vi "convert to TDMS.vi"(7 "defrag?":bool=TRUE, 8 "error in":errorcluster, 11 "path":path) -> (0 "error out":errorcluster)   [LabVIEW 2013, in "Binary datalogger runtime.lvclass"]
uses:
  Binary datalogger runtime.lvclass
  <vilib>/NI/Tag Bus/tag/count types.vi
  <vilib>/NI/Tag Bus/tag/index to type.vi
  <vilib>/NI/Tag Bus/tag/tag descriptor.lvclass
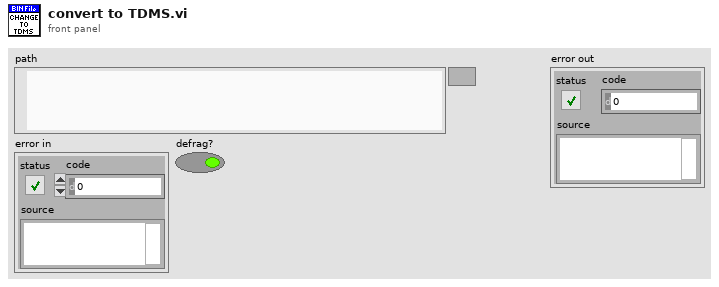
[diagram p1: front panel]
types:
  T1 = typedef "Binary datalogger runtime.lvclass/data cache.ctl" = cluster{"timestamps":timestamp[], "dataset":T2[]}
  T2 = typedef "tag bus.lvlib/data table.lvlib/data table.ctl" = cluster{"Double":dbl[], "Single":sgl[], "I64":i64[], "I32":i32[], "I16":i16[], "I8":i8[], "U64":u64[], "U32":u32[], "U16":u16[], "U8":u8[], "Boolean":bool[], "String":string[], "Array of Double":cluster{"DBL Array":dbl[]}[], "Array of Single":cluster{"SGL Array":sgl[]}[], "Array of I64":cluster{"I64 Array":i64[]}[], "Array of I32":cluster{"I32 Array":i32[]}[], "Array of I16":cluster{"I16 Array":i16[]}[], "Array of I8":cluster{"I8 Array":i8[]}[], "Array of U64":cluster{"U64 Array":u64[]}[], "Array of U32":cluster{"U32 Array":u32[]}[], "Array of U16":cluster{"U16 Array":u16[]}[], "Array of U8":cluster{"U8 Array":u8[]}[], "Array of Boolean":cluster{"Boolean Array":bool[]}[], "Array of String":cluster{"String Array":string[]}[]}
  T3 = typedef "tag bus.lvlib/data dictionary.lvclass/full data dictionary.ctl" = cluster{"Double":string[], "Single":string[], "I64":string[], "I32":string[], "I16":string[], "I8":string[], "U64":string[], "U32":string[], "U16":string[], "U8":string[], "Boolean":string[], "String":string[], "Array of Double":string[], "Array of Single":string[], "Array of I64":string[], "Array of I32":string[], "Array of I16":string[], "Array of I8":string[], "Array of U64":string[], "Array of U32":string[], "Array of U16":string[], "Array of U8":string[], "Array of Boolean":string[], "Array of String":string[]}
  T4 = enum16{"open", "open or create", "create or replace", "create", "open (read-only)"}
  T5 = typedef "tag bus.lvlib/tag descriptor.lvclass/Data Type.ctl" = enum16{"Double", "Single", "I64", "I32", "I16", "I8", "U64", "U32", "U16", "U8", "Boolean", "String", "Array of Double", "Array of Single", "Array of I64", "Array of I32", "Array of I16", "Array of I8", "Array of U64", "Array of U32", "Array of U16", "Array of U8", "Array of Boolean", "Array of String"}
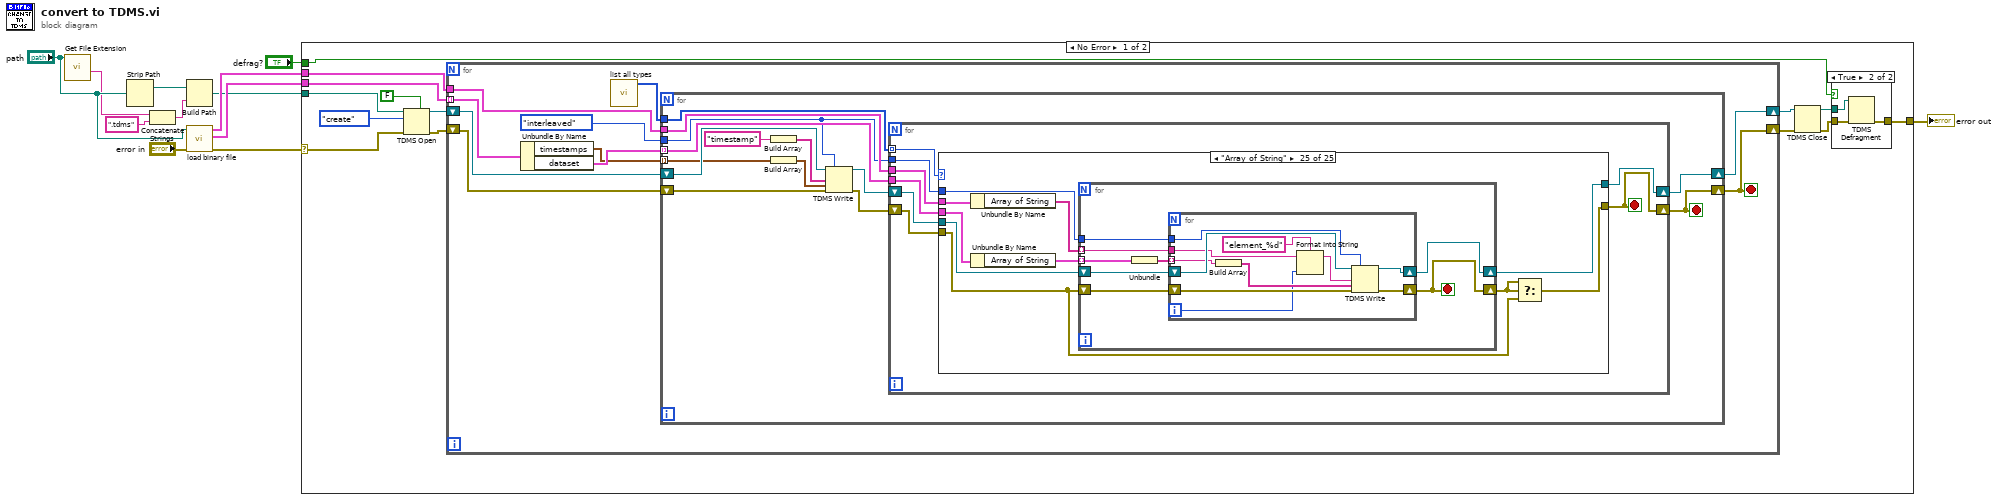
[diagram p0: block diagram]
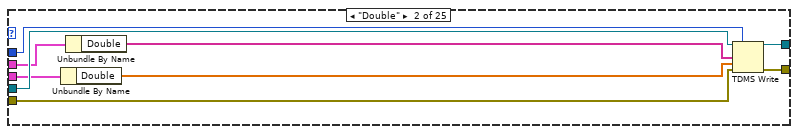
[diagram p3: hidden frame]
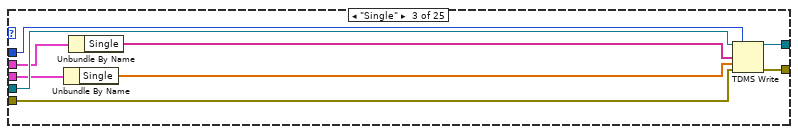
[diagram p4: hidden frame]
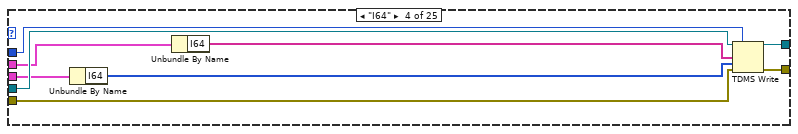
[diagram p5: hidden frame]
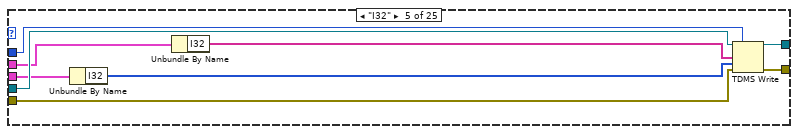
[diagram p6: hidden frame]
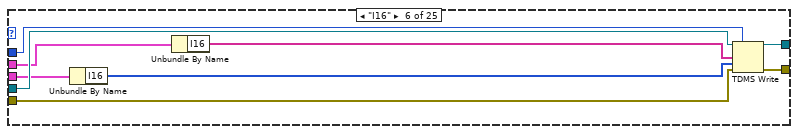
[diagram p7: hidden frame]
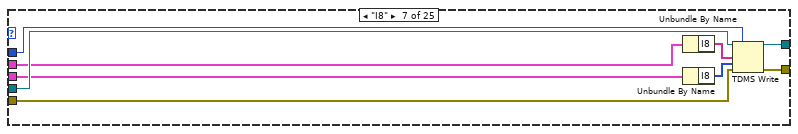
[diagram p8: hidden frame]
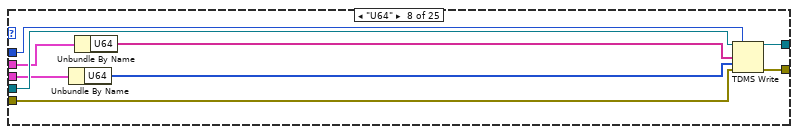
[diagram p9: hidden frame]
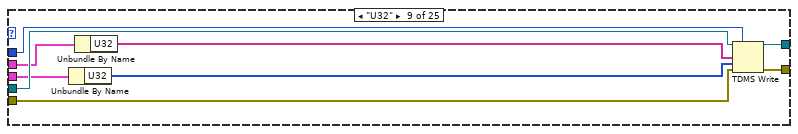
[diagram p10: hidden frame]
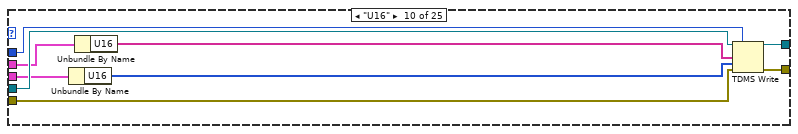
[diagram p11: hidden frame]
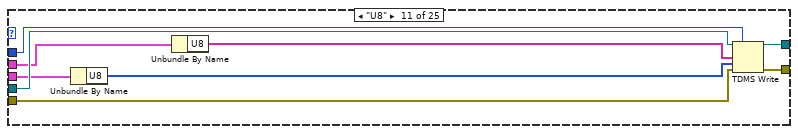
[diagram p12: hidden frame]
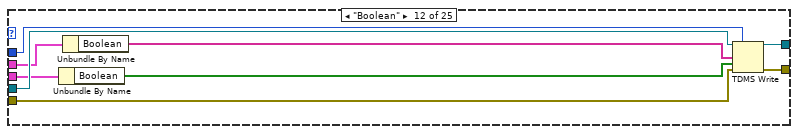
[diagram p13: hidden frame]
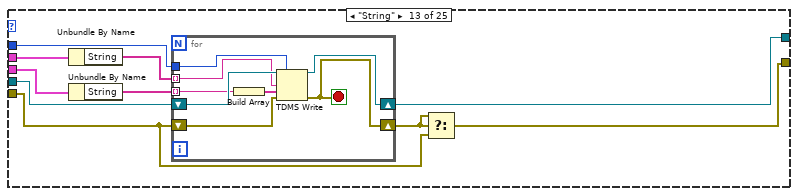
[diagram p14: hidden frame]
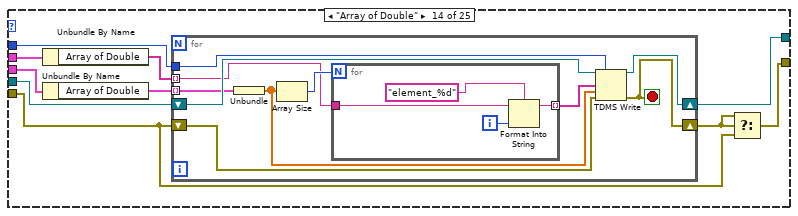
[diagram p15: hidden frame]
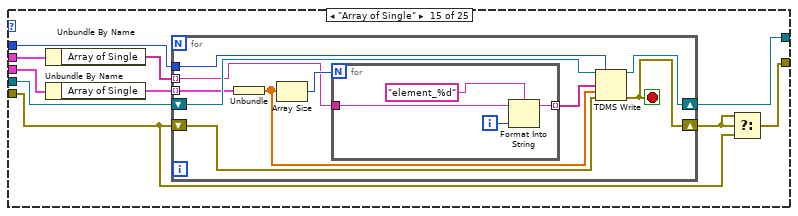
[diagram p16: hidden frame]
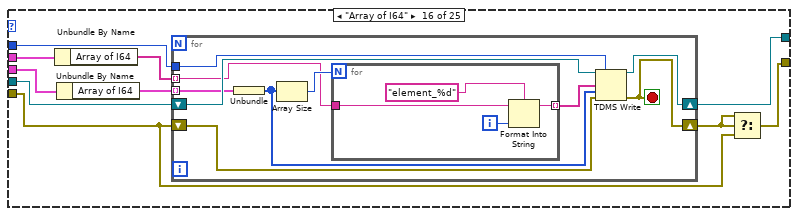
[diagram p17: hidden frame]
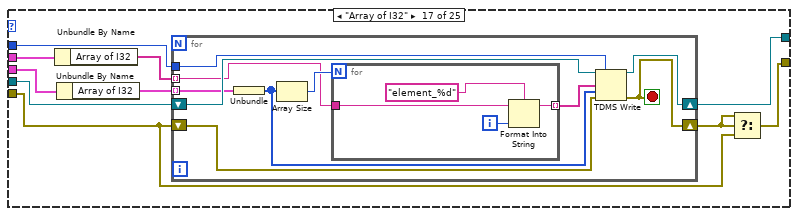
[diagram p18: hidden frame]
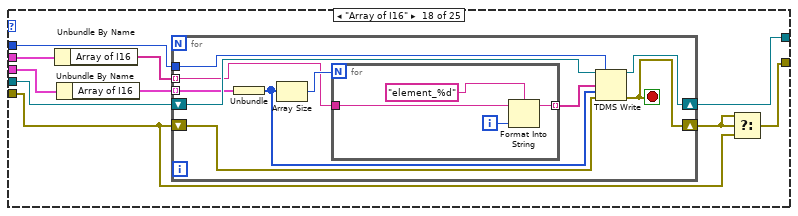
[diagram p19: hidden frame]
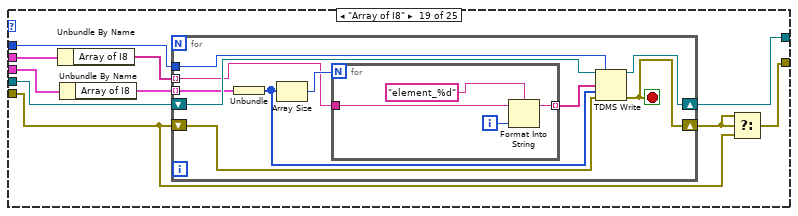
[diagram p20: hidden frame]
diagram:
  n1 = call <vilib>:"Get File Extension.vi"("file"="path") -> ("filename without extension"=w6:string)  [unwired: 7 in, 3 out]
  n2 = Strip Path(path="path") -> (stripped path=w4:path)  [unwired: 1 out]
  n3 = Concatenate Strings(w6, ".tdms" ("string")) -> (w3:string)
  n4 = Build Path(base path=w4, name or relative path=w3) -> (appended path=w2:path)
  n5 = call "load binary file.vi"("error in"="error in", "path"="path") -> ("error out"=w11:errorcluster, "data"=w9:T1[], "dictionary"=w8:T3)  [unwired: 5 in, 2 out]
  n6 = case shown="No Error" w11 {
    selector: w11 -> [w26 w475]
    tunnel: [w21 w475] -> w10
    tunnel: w9 -> [w14 _]
    tunnel: w8 -> [w13 _]
    tunnel: w2 -> [w25 _]
    tunnel: "defrag?" -> [w19 _]
    frame No Error {
      n7 = TDMS Open(5:FALSE ("create index file? (T)"), 8:w26, 10:T4."create" ("operation (0:open)"), 11:w25) -> (0:w16:errorcluster, 3:w18:refnum<k34>)  [unwired: 3 in]
      n8 = for {
        shift-right: [w36] -> w17
        shift-left: w18 -> [w30]
        shift-right: [w35] -> w15
        shift-left: w16 -> [w31]
        tunnel: w14 -> [w34] mode=indexing
        tunnel: w13 -> [w32]
        stop <- w35 stop-if-true
        n9 = Unbundle By Name(w34) -> ("timestamps"=w27:timestamp[], "dataset"=w33:T2[])
        n10 = call <vilib>:"list all types.vi"() -> ("all types"=w29:T5[])  [unwired: 11 in]
        n11 = for {
          shift-right: [w49] -> w36
          shift-left: w30 -> [w43]
          shift-right: [w45] -> w35
          shift-left: w31 -> [w48]
          tunnel: w33 -> [w46] mode=indexing
          tunnel: w32 -> [w47]
          tunnel: w29 -> [w50]
          tunnel: enum16{"decimated", "interleaved"}."interleaved" ("data layout (0:decimated)") -> [w41]
          tunnel: w27 -> [w38] mode=indexing
          stop <- w45 stop-if-true
          n12 = Build Array("timestamp") -> (w39:string[])
          n13 = Build Array(w38) -> (w37:timestamp[])
          n14 = TDMS Write(0:w43, 1:w41, 7:w39, 9:w37, 11:w48) -> (4:w42:refnum<k34>, 15:w44:errorcluster)  [unwired: 1 in, 2 out]
          n15 = for {
            tunnel: w50 -> [w58] mode=indexing
            tunnel: w47 -> [w54]
            tunnel: w46 -> [w53]
            tunnel: w41 -> [w52]
            shift-right: [w57] -> w49
            shift-left: w42 -> [w56]
            shift-right: [w51] -> w45
            shift-left: w44 -> [w55]
            stop <- w51 stop-if-true
            n16 = case shown="\"Array of String\"" w58 {
              tunnel: [w60 w66 w75 w84 w93 w102 w111 w120 w129 w138 w147 w156 w168 w186 w210 w234 w258 w282 w306 w330 w354 w378 w402 w426 w450] -> w57
              tunnel: w56 -> [w60 w69 w78 w87 w96 w105 w114 w123 w132 w141 w150 w159 w169 w187 w211 w235 w259 w283 w307 w331 w355 w379 w403 w427 w451]
              tunnel: w55 -> [w59 w68 w77 w86 w95 w104 w113 w122 w131 w140 w149 w158 w161 w179 w203 w227 w251 w275 w299 w323 w347 w371 w395 w419 w443]
              tunnel: [w59 w67 w76 w85 w94 w103 w112 w121 w130 w139 w148 w157 w160 w178 w202 w226 w250 w274 w298 w322 w346 w370 w394 w418 w442] -> w51
              tunnel: w54 -> [_ w65 w74 w83 w92 w101 w110 w119 w128 w137 w146 w155 w167 w185 w209 w233 w257 w281 w305 w329 w353 w377 w401 w425 w449]
              tunnel: w53 -> [_ w64 w73 w82 w91 w100 w109 w118 w127 w136 w145 w154 w166 w184 w208 w232 w256 w280 w304 w328 w352 w376 w400 w424 w448]
              tunnel: w52 -> [_ w61 w70 w79 w88 w97 w106 w115 w124 w133 w142 w151 w163 w181 w205 w229 w253 w277 w301 w325 w349 w373 w397 w421 w445]
              frame Default {
              }
              frame "Double" {
                n17 = Unbundle By Name(w64) -> ("Double"=w63:dbl[])
                n18 = Unbundle By Name(w65) -> ("Double"=w62:string[])
                n19 = TDMS Write(0:w69, 1:w61, 7:w62, 9:w63, 11:w68) -> (4:w66:refnum<k34>, 15:w67:errorcluster)  [unwired: 1 in, 2 out]
              }
              frame "Single" {
                n20 = Unbundle By Name(w73) -> ("Single"=w72:sgl[])
                n21 = Unbundle By Name(w74) -> ("Single"=w71:string[])
                n22 = TDMS Write(0:w78, 1:w70, 7:w71, 9:w72, 11:w77) -> (4:w75:refnum<k34>, 15:w76:errorcluster)  [unwired: 1 in, 2 out]
              }
              frame "I64" {
                n23 = Unbundle By Name(w82) -> ("I64"=w81:i64[])
                n24 = Unbundle By Name(w83) -> ("I64"=w80:string[])
                n25 = TDMS Write(0:w87, 1:w79, 7:w80, 9:w81, 11:w86) -> (4:w84:refnum<k34>, 15:w85:errorcluster)  [unwired: 1 in, 2 out]
              }
              frame "I32" {
                n26 = Unbundle By Name(w91) -> ("I32"=w90:i32[])
                n27 = Unbundle By Name(w92) -> ("I32"=w89:string[])
                n28 = TDMS Write(0:w96, 1:w88, 7:w89, 9:w90, 11:w95) -> (4:w93:refnum<k34>, 15:w94:errorcluster)  [unwired: 1 in, 2 out]
              }
              frame "I16" {
                n29 = Unbundle By Name(w100) -> ("I16"=w99:i16[])
                n30 = Unbundle By Name(w101) -> ("I16"=w98:string[])
                n31 = TDMS Write(0:w105, 1:w97, 7:w98, 9:w99, 11:w104) -> (4:w102:refnum<k34>, 15:w103:errorcluster)  [unwired: 1 in, 2 out]
              }
              frame "I8" {
                n32 = Unbundle By Name(w110) -> ("I8"=w107:string[])
                n33 = Unbundle By Name(w109) -> ("I8"=w108:i8[])
                n34 = TDMS Write(0:w114, 1:w106, 7:w107, 9:w108, 11:w113) -> (4:w111:refnum<k34>, 15:w112:errorcluster)  [unwired: 1 in, 2 out]
              }
              frame "U64" {
                n35 = Unbundle By Name(w118) -> ("U64"=w117:u64[])
                n36 = Unbundle By Name(w119) -> ("U64"=w116:string[])
                n37 = TDMS Write(0:w123, 1:w115, 7:w116, 9:w117, 11:w122) -> (4:w120:refnum<k34>, 15:w121:errorcluster)  [unwired: 1 in, 2 out]
              }
              frame "U32" {
                n38 = Unbundle By Name(w127) -> ("U32"=w126:u32[])
                n39 = Unbundle By Name(w128) -> ("U32"=w125:string[])
                n40 = TDMS Write(0:w132, 1:w124, 7:w125, 9:w126, 11:w131) -> (4:w129:refnum<k34>, 15:w130:errorcluster)  [unwired: 1 in, 2 out]
              }
              frame "U16" {
                n41 = Unbundle By Name(w136) -> ("U16"=w135:u16[])
                n42 = Unbundle By Name(w137) -> ("U16"=w134:string[])
                n43 = TDMS Write(0:w141, 1:w133, 7:w134, 9:w135, 11:w140) -> (4:w138:refnum<k34>, 15:w139:errorcluster)  [unwired: 1 in, 2 out]
              }
              frame "U8" {
                n44 = Unbundle By Name(w145) -> ("U8"=w144:u8[])
                n45 = Unbundle By Name(w146) -> ("U8"=w143:string[])
                n46 = TDMS Write(0:w150, 1:w142, 7:w143, 9:w144, 11:w149) -> (4:w147:refnum<k34>, 15:w148:errorcluster)  [unwired: 1 in, 2 out]
              }
              frame "Boolean" {
                n47 = Unbundle By Name(w154) -> ("Boolean"=w153:bool[])
                n48 = Unbundle By Name(w155) -> ("Boolean"=w152:string[])
                n49 = TDMS Write(0:w159, 1:w151, 7:w152, 9:w153, 11:w158) -> (4:w156:refnum<k34>, 15:w157:errorcluster)  [unwired: 1 in, 2 out]
              }
              frame "String" {
                n50 = Unbundle By Name(w167) -> ("String"=w164:string[])
                n51 = Unbundle By Name(w166) -> ("String"=w165:string[])
                n52 = for {
                  tunnel: w165 -> [w174] mode=indexing
                  tunnel: w164 -> [w172] mode=indexing
                  tunnel: w163 -> [w173]
                  shift-right: [w175] -> w168
                  shift-left: w169 -> [w177]
                  shift-right: [w170] -> w162
                  shift-left: w161 -> [w176]
                  stop <- w170 stop-if-true
                  n53 = Build Array(w174) -> (w171:string[])
                  n54 = TDMS Write(0:w177, 1:w173, 7:w172, 9:w171, 11:w176) -> (4:w175:refnum<k34>, 15:w170:errorcluster)  [unwired: 1 in, 2 out]
                }
                n55 = Select(t=w162, s=w162, f=w161) -> (s? t:f=w160:errorcluster)
              }
              frame "Array of Double" {
                n56 = Unbundle By Name(w185) -> ("Array of Double"=w182:string[])
                n57 = Unbundle By Name(w184) -> ("Array of Double"=w183:cluster{"DBL Array":dbl[]}[])
                n58 = for {
                  tunnel: w183 -> [w192] mode=indexing
                  tunnel: w182 -> [w189] mode=indexing
                  tunnel: w181 -> [w194]
                  shift-right: [w195] -> w186
                  shift-left: w187 -> [w197]
                  shift-right: [w193] -> w180
                  shift-left: w179 -> [w196]
                  stop <- w193 stop-if-true
                  n59 = Unbundle(w192) -> ("DBL Array"=w191:dbl[])
                  n60 = Array Size(array=w191) -> (size(s)=w190:i32)
                  n61 = for {
                    N: w190 -> [_]
                    tunnel: w189 -> [w201]
                    tunnel: [w198] -> w188 mode=indexing
                    i -> [w200]
                    n62 = Format Into String(format string="element_%d", initial string=w201, w200) -> (resulting string=w198:string)  [unwired: 1 in, 1 out]
                  }
                  n63 = TDMS Write(0:w197, 1:w194, 7:w188, 9:w191, 11:w196) -> (4:w195:refnum<k34>, 15:w193:errorcluster)  [unwired: 1 in, 2 out]
                }
                n64 = Select(t=w180, s=w180, f=w179) -> (s? t:f=w178:errorcluster)
              }
              frame "Array of Single" {
                n65 = Unbundle By Name(w209) -> ("Array of Single"=w206:string[])
                n66 = Unbundle By Name(w208) -> ("Array of Single"=w207:cluster{"SGL Array":sgl[]}[])
                n67 = for {
                  tunnel: w207 -> [w216] mode=indexing
                  tunnel: w206 -> [w213] mode=indexing
                  tunnel: w205 -> [w218]
                  shift-right: [w219] -> w210
                  shift-left: w211 -> [w221]
                  shift-right: [w217] -> w204
                  shift-left: w203 -> [w220]
                  stop <- w217 stop-if-true
                  n68 = Unbundle(w216) -> ("SGL Array"=w215:sgl[])
                  n69 = Array Size(array=w215) -> (size(s)=w214:i32)
                  n70 = for {
                    N: w214 -> [_]
                    tunnel: w213 -> [w225]
                    tunnel: [w222] -> w212 mode=indexing
                    i -> [w224]
                    n71 = Format Into String(format string="element_%d", initial string=w225, w224) -> (resulting string=w222:string)  [unwired: 1 in, 1 out]
                  }
                  n72 = TDMS Write(0:w221, 1:w218, 7:w212, 9:w215, 11:w220) -> (4:w219:refnum<k34>, 15:w217:errorcluster)  [unwired: 1 in, 2 out]
                }
                n73 = Select(t=w204, s=w204, f=w203) -> (s? t:f=w202:errorcluster)
              }
              frame "Array of I64" {
                n74 = Unbundle By Name(w233) -> ("Array of I64"=w230:string[])
                n75 = Unbundle By Name(w232) -> ("Array of I64"=w231:cluster{"I64 Array":i64[]}[])
                n76 = for {
                  tunnel: w231 -> [w240] mode=indexing
                  tunnel: w230 -> [w237] mode=indexing
                  tunnel: w229 -> [w242]
                  shift-right: [w243] -> w234
                  shift-left: w235 -> [w245]
                  shift-right: [w241] -> w228
                  shift-left: w227 -> [w244]
                  stop <- w241 stop-if-true
                  n77 = Unbundle(w240) -> ("I64 Array"=w239:i64[])
                  n78 = Array Size(array=w239) -> (size(s)=w238:i32)
                  n79 = for {
                    N: w238 -> [_]
                    tunnel: w237 -> [w249]
                    tunnel: [w246] -> w236 mode=indexing
                    i -> [w248]
                    n80 = Format Into String(format string="element_%d", initial string=w249, w248) -> (resulting string=w246:string)  [unwired: 1 in, 1 out]
                  }
                  n81 = TDMS Write(0:w245, 1:w242, 7:w236, 9:w239, 11:w244) -> (4:w243:refnum<k34>, 15:w241:errorcluster)  [unwired: 1 in, 2 out]
                }
                n82 = Select(t=w228, s=w228, f=w227) -> (s? t:f=w226:errorcluster)
              }
              frame "Array of I32" {
                n83 = Unbundle By Name(w257) -> ("Array of I32"=w254:string[])
                n84 = Unbundle By Name(w256) -> ("Array of I32"=w255:cluster{"I32 Array":i32[]}[])
                n85 = for {
                  tunnel: w255 -> [w264] mode=indexing
                  tunnel: w254 -> [w261] mode=indexing
                  tunnel: w253 -> [w266]
                  shift-right: [w267] -> w258
                  shift-left: w259 -> [w269]
                  shift-right: [w265] -> w252
                  shift-left: w251 -> [w268]
                  stop <- w265 stop-if-true
                  n86 = Unbundle(w264) -> ("I32 Array"=w263:i32[])
                  n87 = Array Size(array=w263) -> (size(s)=w262:i32)
                  n88 = for {
                    N: w262 -> [_]
                    tunnel: w261 -> [w273]
                    tunnel: [w270] -> w260 mode=indexing
                    i -> [w272]
                    n89 = Format Into String(format string="element_%d", initial string=w273, w272) -> (resulting string=w270:string)  [unwired: 1 in, 1 out]
                  }
                  n90 = TDMS Write(0:w269, 1:w266, 7:w260, 9:w263, 11:w268) -> (4:w267:refnum<k34>, 15:w265:errorcluster)  [unwired: 1 in, 2 out]
                }
                n91 = Select(t=w252, s=w252, f=w251) -> (s? t:f=w250:errorcluster)
              }
              frame "Array of I16" {
                n92 = Unbundle By Name(w281) -> ("Array of I16"=w278:string[])
                n93 = Unbundle By Name(w280) -> ("Array of I16"=w279:cluster{"I16 Array":i16[]}[])
                n94 = for {
                  tunnel: w279 -> [w288] mode=indexing
                  tunnel: w278 -> [w285] mode=indexing
                  tunnel: w277 -> [w290]
                  shift-right: [w291] -> w282
                  shift-left: w283 -> [w293]
                  shift-right: [w289] -> w276
                  shift-left: w275 -> [w292]
                  stop <- w289 stop-if-true
                  n95 = Unbundle(w288) -> ("I16 Array"=w287:i16[])
                  n96 = Array Size(array=w287) -> (size(s)=w286:i32)
                  n97 = for {
                    N: w286 -> [_]
                    tunnel: w285 -> [w297]
                    tunnel: [w294] -> w284 mode=indexing
                    i -> [w296]
                    n98 = Format Into String(format string="element_%d", initial string=w297, w296) -> (resulting string=w294:string)  [unwired: 1 in, 1 out]
                  }
                  n99 = TDMS Write(0:w293, 1:w290, 7:w284, 9:w287, 11:w292) -> (4:w291:refnum<k34>, 15:w289:errorcluster)  [unwired: 1 in, 2 out]
                }
                n100 = Select(t=w276, s=w276, f=w275) -> (s? t:f=w274:errorcluster)
              }
              frame "Array of I8" {
                n101 = Unbundle By Name(w305) -> ("Array of I8"=w302:string[])
                n102 = Unbundle By Name(w304) -> ("Array of I8"=w303:cluster{"I8 Array":i8[]}[])
                n103 = for {
                  tunnel: w303 -> [w312] mode=indexing
                  tunnel: w302 -> [w309] mode=indexing
                  tunnel: w301 -> [w314]
                  shift-right: [w315] -> w306
                  shift-left: w307 -> [w317]
                  shift-right: [w313] -> w300
                  shift-left: w299 -> [w316]
                  stop <- w313 stop-if-true
                  n104 = Unbundle(w312) -> ("I8 Array"=w311:i8[])
                  n105 = Array Size(array=w311) -> (size(s)=w310:i32)
                  n106 = for {
                    N: w310 -> [_]
                    tunnel: w309 -> [w321]
                    tunnel: [w318] -> w308 mode=indexing
                    i -> [w320]
                    n107 = Format Into String(format string="element_%d", initial string=w321, w320) -> (resulting string=w318:string)  [unwired: 1 in, 1 out]
                  }
                  n108 = TDMS Write(0:w317, 1:w314, 7:w308, 9:w311, 11:w316) -> (4:w315:refnum<k34>, 15:w313:errorcluster)  [unwired: 1 in, 2 out]
                }
                n109 = Select(t=w300, s=w300, f=w299) -> (s? t:f=w298:errorcluster)
              }
              frame "Array of U64" {
                n110 = Unbundle By Name(w329) -> ("Array of U64"=w326:string[])
                n111 = Unbundle By Name(w328) -> ("Array of U64"=w327:cluster{"U64 Array":u64[]}[])
                n112 = for {
                  tunnel: w327 -> [w336] mode=indexing
                  tunnel: w326 -> [w333] mode=indexing
                  tunnel: w325 -> [w338]
                  shift-right: [w339] -> w330
                  shift-left: w331 -> [w341]
                  shift-right: [w337] -> w324
                  shift-left: w323 -> [w340]
                  stop <- w337 stop-if-true
                  n113 = Unbundle(w336) -> ("U64 Array"=w335:u64[])
                  n114 = Array Size(array=w335) -> (size(s)=w334:i32)
                  n115 = for {
                    N: w334 -> [_]
                    tunnel: w333 -> [w345]
                    tunnel: [w342] -> w332 mode=indexing
                    i -> [w344]
                    n116 = Format Into String(format string="element_%d", initial string=w345, w344) -> (resulting string=w342:string)  [unwired: 1 in, 1 out]
                  }
                  n117 = TDMS Write(0:w341, 1:w338, 7:w332, 9:w335, 11:w340) -> (4:w339:refnum<k34>, 15:w337:errorcluster)  [unwired: 1 in, 2 out]
                }
                n118 = Select(t=w324, s=w324, f=w323) -> (s? t:f=w322:errorcluster)
              }
              frame "Array of U32" {
                n119 = Unbundle By Name(w353) -> ("Array of U32"=w350:string[])
                n120 = Unbundle By Name(w352) -> ("Array of U32"=w351:cluster{"U32 Array":u32[]}[])
                n121 = for {
                  tunnel: w351 -> [w360] mode=indexing
                  tunnel: w350 -> [w357] mode=indexing
                  tunnel: w349 -> [w362]
                  shift-right: [w363] -> w354
                  shift-left: w355 -> [w365]
                  shift-right: [w361] -> w348
                  shift-left: w347 -> [w364]
                  stop <- w361 stop-if-true
                  n122 = Unbundle(w360) -> ("U32 Array"=w359:u32[])
                  n123 = Array Size(array=w359) -> (size(s)=w358:i32)
                  n124 = for {
                    N: w358 -> [_]
                    tunnel: w357 -> [w369]
                    tunnel: [w366] -> w356 mode=indexing
                    i -> [w368]
                    n125 = Format Into String(format string="element_%d", initial string=w369, w368) -> (resulting string=w366:string)  [unwired: 1 in, 1 out]
                  }
                  n126 = TDMS Write(0:w365, 1:w362, 7:w356, 9:w359, 11:w364) -> (4:w363:refnum<k34>, 15:w361:errorcluster)  [unwired: 1 in, 2 out]
                }
                n127 = Select(t=w348, s=w348, f=w347) -> (s? t:f=w346:errorcluster)
              }
              frame "Array of U16" {
                n128 = Unbundle By Name(w377) -> ("Array of U16"=w374:string[])
                n129 = Unbundle By Name(w376) -> ("Array of U16"=w375:cluster{"U16 Array":u16[]}[])
                n130 = for {
                  tunnel: w375 -> [w384] mode=indexing
                  tunnel: w374 -> [w381] mode=indexing
                  tunnel: w373 -> [w386]
                  shift-right: [w387] -> w378
                  shift-left: w379 -> [w389]
                  shift-right: [w385] -> w372
                  shift-left: w371 -> [w388]
                  stop <- w385 stop-if-true
                  n131 = Unbundle(w384) -> ("U16 Array"=w383:u16[])
                  n132 = Array Size(array=w383) -> (size(s)=w382:i32)
                  n133 = for {
                    N: w382 -> [_]
                    tunnel: w381 -> [w393]
                    tunnel: [w390] -> w380 mode=indexing
                    i -> [w392]
                    n134 = Format Into String(format string="element_%d", initial string=w393, w392) -> (resulting string=w390:string)  [unwired: 1 in, 1 out]
                  }
                  n135 = TDMS Write(0:w389, 1:w386, 7:w380, 9:w383, 11:w388) -> (4:w387:refnum<k34>, 15:w385:errorcluster)  [unwired: 1 in, 2 out]
                }
                n136 = Select(t=w372, s=w372, f=w371) -> (s? t:f=w370:errorcluster)
              }
              frame "Array of U8" {
                n137 = Unbundle By Name(w401) -> ("Array of U8"=w398:string[])
                n138 = Unbundle By Name(w400) -> ("Array of U8"=w399:cluster{"U8 Array":u8[]}[])
                n139 = for {
                  tunnel: w399 -> [w408] mode=indexing
                  tunnel: w398 -> [w405] mode=indexing
                  tunnel: w397 -> [w410]
                  shift-right: [w411] -> w402
                  shift-left: w403 -> [w413]
                  shift-right: [w409] -> w396
                  shift-left: w395 -> [w412]
                  stop <- w409 stop-if-true
                  n140 = Unbundle(w408) -> ("U8 Array"=w407:u8[])
                  n141 = Array Size(array=w407) -> (size(s)=w406:i32)
                  n142 = for {
                    N: w406 -> [_]
                    tunnel: w405 -> [w417]
                    tunnel: [w414] -> w404 mode=indexing
                    i -> [w416]
                    n143 = Format Into String(format string="element_%d", initial string=w417, w416) -> (resulting string=w414:string)  [unwired: 1 in, 1 out]
                  }
                  n144 = TDMS Write(0:w413, 1:w410, 7:w404, 9:w407, 11:w412) -> (4:w411:refnum<k34>, 15:w409:errorcluster)  [unwired: 1 in, 2 out]
                }
                n145 = Select(t=w396, s=w396, f=w395) -> (s? t:f=w394:errorcluster)
              }
              frame "Array of Boolean" {
                n146 = Unbundle By Name(w425) -> ("Array of Boolean"=w422:string[])
                n147 = Unbundle By Name(w424) -> ("Array of Boolean"=w423:cluster{"Boolean Array":bool[]}[])
                n148 = for {
                  tunnel: w423 -> [w432] mode=indexing
                  tunnel: w422 -> [w429] mode=indexing
                  tunnel: w421 -> [w434]
                  shift-right: [w435] -> w426
                  shift-left: w427 -> [w437]
                  shift-right: [w433] -> w420
                  shift-left: w419 -> [w436]
                  stop <- w433 stop-if-true
                  n149 = Unbundle(w432) -> ("Boolean Array"=w431:bool[])
                  n150 = Array Size(array=w431) -> (size(s)=w430:i32)
                  n151 = for {
                    N: w430 -> [_]
                    tunnel: w429 -> [w441]
                    tunnel: [w438] -> w428 mode=indexing
                    i -> [w440]
                    n152 = Format Into String(format string="element_%d", initial string=w441, w440) -> (resulting string=w438:string)  [unwired: 1 in, 1 out]
                  }
                  n153 = TDMS Write(0:w437, 1:w434, 7:w428, 9:w431, 11:w436) -> (4:w435:refnum<k34>, 15:w433:errorcluster)  [unwired: 1 in, 2 out]
                }
                n154 = Select(t=w420, s=w420, f=w419) -> (s? t:f=w418:errorcluster)
              }
              frame "Array of String" {
                n155 = Unbundle By Name(w449) -> ("Array of String"=w446:string[])
                n156 = Unbundle By Name(w448) -> ("Array of String"=w447:cluster{"String Array":string[]}[])
                n157 = for {
                  tunnel: w447 -> [w454] mode=indexing
                  tunnel: w446 -> [w452] mode=indexing
                  tunnel: w445 -> [w456]
                  shift-right: [w457] -> w450
                  shift-left: w451 -> [w459]
                  shift-right: [w455] -> w444
                  shift-left: w443 -> [w458]
                  stop <- w455 stop-if-true
                  n158 = Unbundle(w454) -> ("String Array"=w453:string[])
                  n159 = for {
                    tunnel: w456 -> [w467]
                    tunnel: w453 -> [w465] mode=indexing
                    tunnel: w452 -> [w464]
                    shift-right: [w468] -> w457
                    shift-left: w459 -> [w470]
                    shift-right: [w466] -> w455
                    shift-left: w458 -> [w469]
                    i -> [w460]
                    n160 = Build Array(w465) -> (w461:string[])
                    n161 = Format Into String(format string="element_%d", initial string=w464, w460) -> (resulting string=w463:string)  [unwired: 1 in, 1 out]
                    n162 = TDMS Write(0:w470, 1:w467, 7:w463, 9:w461, 11:w469) -> (4:w468:refnum<k34>, 15:w466:errorcluster)  [unwired: 1 in, 2 out]
                  }
                }
                n163 = Select(t=w444, s=w444, f=w443) -> (s? t:f=w442:errorcluster)
              }
            }
          }
        }
      }
      n164 = TDMS Close(8:w15, 11:w17) -> (0:w22:errorcluster, 3:w20:path)
      n165 = case shown="True" w19 {
        tunnel: w22 -> [w471 w474]
        tunnel: [w471 w473] -> w21
        tunnel: w20 -> [_ w472]
        frame False {
        }
        frame True {
          n166 = TDMS Defragment(4:w474, 7:w472) -> (0:w473:errorcluster)
        }
      }
    }
    frame Error {
    }
  }
  "error out" <- w10
